vi "AmpScan TestCode2.vi"() -> ()   [LabVIEW 2018]
panel:
  out "Waveform Graph":dbl[](graph)
  in  "MaxAmp":ext
  in  "AuxPulses":ext[](array[numeric])
  in  "Amp":ext[](array[numeric])
  in  "AuxAmp":ext[](array[numeric])
  out "Amp2":ext
  in  "Scan time":ext
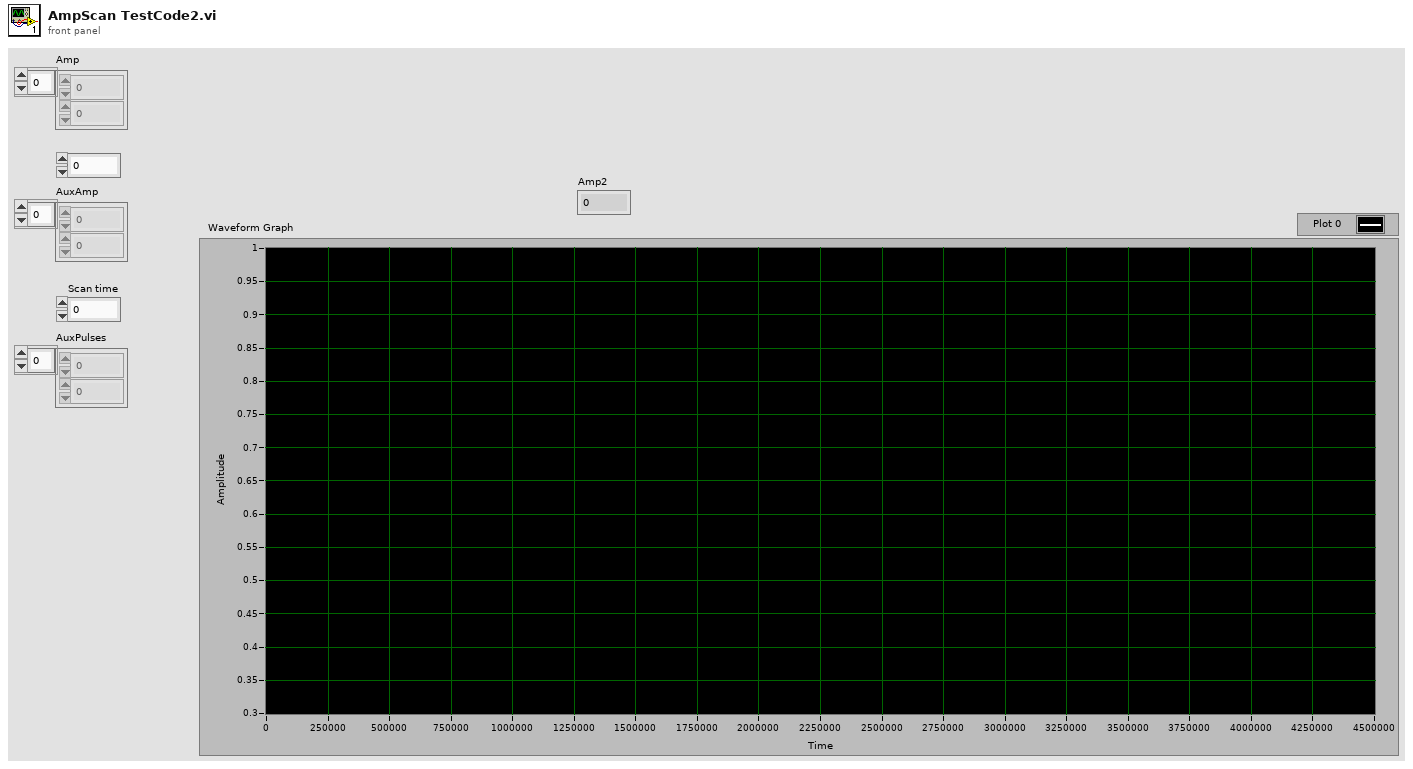
[diagram p1: front panel]
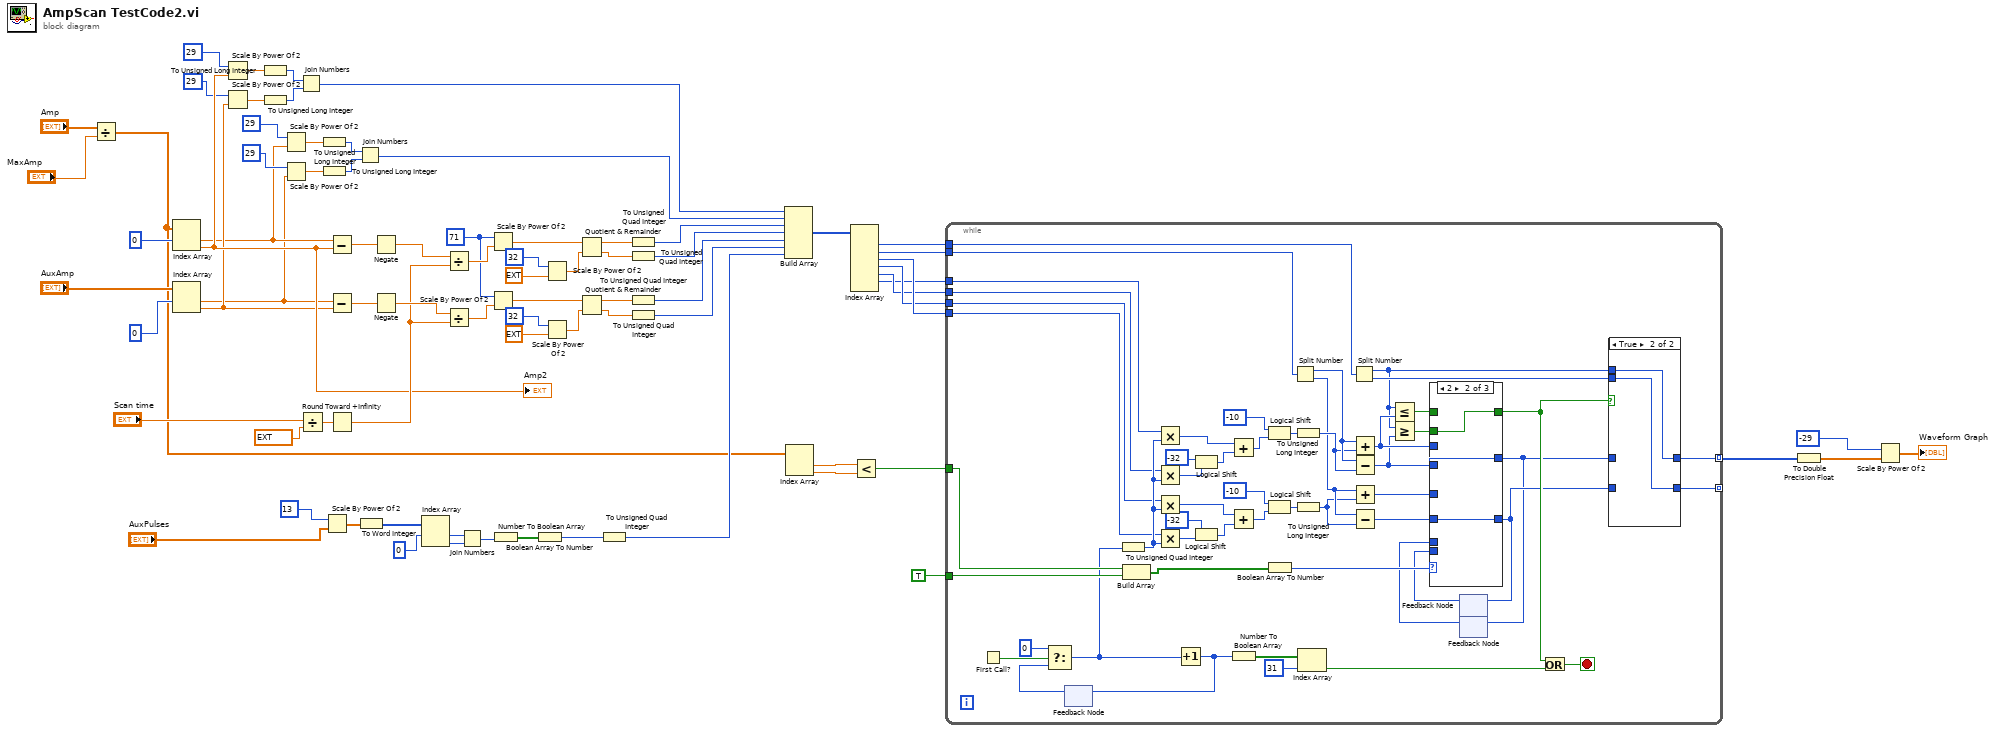
[diagram p0: block diagram]
diagram:
  w65 = i16 71 ("n")
  n1 = Divide(x="Amp", y="MaxAmp") -> (x/y=w7:ext[])
  n2 = Index Array(array=w7, index #1=0 ("index")) -> (element #1=w20:ext, element #2=w33:ext)  [unwired: 1 in]
  "Amp2" <- w33
  n3 = Index Array(array="AuxAmp", index #1=0 ("index")) -> (element #1=w19:ext, element #2=w30:ext)  [unwired: 1 in]
  n4 = Scale By Power Of 2(n=i16 29, x=w33) -> (x*2^n=w61:ext)
  n5 = Scale By Power Of 2(n=i16 29, x=w30) -> (x*2^n=w32:ext)
  n6 = To Unsigned Long Integer(number=w61) -> (unsigned 32bit integer=w29:u32)
  n7 = To Unsigned Long Integer(number=w32) -> (unsigned 32bit integer=w28:u32)
  n8 = Scale By Power Of 2(n=i16 29, x=w20) -> (x*2^n=w22:ext)
  n9 = Scale By Power Of 2(n=i16 29, x=w19) -> (x*2^n=w23:ext)
  n10 = Join Numbers(hi=w29, lo=w28) -> ((hi.lo)=w27:u64)
  n11 = Divide(x="Scan time", y=ext 2.5e-08) -> (x/y=w72:ext)
  n12 = To Unsigned Long Integer(number=w22) -> (unsigned 32bit integer=w25:u32)
  n13 = To Unsigned Long Integer(number=w23) -> (unsigned 32bit integer=w26:u32)
  n14 = Scale By Power Of 2(n=i16 13, x="AuxPulses") -> (x*2^n=w42:ext[])
  n15 = Subtract(x=w20, y=w33) -> (x-y=w77:ext)
  n16 = Subtract(x=w19, y=w30) -> (x-y=w76:ext)
  n17 = Round Toward +Infinity(x=w72) -> (ceil(x): smallest int >= x=w67:ext)
  n18 = Join Numbers(hi=w25, lo=w26) -> ((hi.lo)=w18:u64)
  n19 = To Word Integer(number=w42) -> (16bit integer=w41:i16[])
  n20 = Negate(x=w77) -> (-x=w62:ext)
  n21 = Negate(x=w76) -> (-x=w75:ext)
  n22 = Index Array(array=w41, index #1=0 ("index")) -> (element #1=w39:i16, element #2=w38:i16)  [unwired: 1 in]
  n23 = Divide(x=w62, y=w67) -> (x/y=w66:ext)
  n24 = Divide(x=w75, y=w67) -> (x/y=w64:ext)
  n25 = Join Numbers(hi=w39, lo=w38) -> ((hi.lo)=w37:u32)
  n26 = Scale By Power Of 2(n=w65, x=w66) -> (x*2^n=w57:ext)
  n27 = Scale By Power Of 2(n=w65, x=w64) -> (x*2^n=w53:ext)
  n28 = Number To Boolean Array(number=w37) -> (Boolean array=w36:bool[])
  n29 = Boolean Array To Number(Boolean array=w36) -> (number=w35:u32)
  n30 = Scale By Power Of 2(n=i16 32, x=ext 1.0) -> (x*2^n=w58:ext)
  n31 = Scale By Power Of 2(n=i16 32, x=ext 1.0) -> (x*2^n=w56:ext)
  n32 = Quotient & Remainder(x=w57, y=w58) -> (x-y*floor(x/y)=w52:ext, floor(x/y)=w50:ext)
  n33 = Quotient & Remainder(x=w53, y=w56) -> (x-y*floor(x/y)=w48:ext, floor(x/y)=w46:ext)
  n34 = To Unsigned Quad Integer(1:w35) -> (0:w34:u64)
  n35 = To Unsigned Quad Integer(1:w52) -> (0:w51:u64)
  n36 = To Unsigned Quad Integer(1:w50) -> (0:w49:u64)
  n37 = To Unsigned Quad Integer(1:w48) -> (0:w47:u64)
  n38 = To Unsigned Quad Integer(1:w46) -> (0:w45:u64)
  n39 = Build Array(w27, w18, w51, w49, w47, w45, w34) -> (w17:u64[])
  n40 = Index Array(array=w7) -> (element #1=w9:ext, element #2=w8:ext)  [unwired: 2 in]
  n41 = Index Array(array=w17) -> (element #1=w16:u64, element #2=w15:u64, element #3=w14:u64, element #4=w13:u64, element #5=w12:u64, element #6=w11:u64)  [unwired: 7 in, 1 out]
  n42 = Less?(x=w9, y=w8) -> (x < y?=w6:bool)
  n43 = while {
    tunnel: w16 -> [w91]
    tunnel: w15 -> [w90]
    tunnel: w14 -> [w86]
    tunnel: w13 -> [w87]
    tunnel: w12 -> [w88]
    tunnel: w11 -> [w89]
    tunnel: w6 -> [w93]
    tunnel: TRUE -> [w92]
    tunnel: [w79] -> w2 mode=indexing
    tunnel: [w78] -> _ mode=indexing
    stop <- w123 stop-if-true
    n44 = First Call?() -> (First Call?: T/F=w128:bool)
    n45 = feedback #1() -> (w129:u32)  [unwired: 1 in]
    n46 = Select(t=u32 0 ("index"), s=w128, f=w129) -> (s? t:f=w85:u32)
    n47 = To Unsigned Quad Integer(1:w85) -> (0:w108:u64)
    n48 = Build Array(w93, w92) -> (w103:bool[])
    n49 = Multiply(x=w89, y=w108) -> (x*y=w122:u64)
    n50 = Multiply(x=w88, y=w108) -> (x*y=w120:u64)
    n51 = Multiply(x=w87, y=w108) -> (x*y=w111:u64)
    n52 = Multiply(x=w86, y=w108) -> (x*y=w110:u64)
    n53 = Increment(x=w85) -> (x+1=w127:u32)
    n54 = feedback-in #1(w127) -> ()
    n55 = Logical Shift(y=i16 -32 ("n"), x=w120) -> (x << y=w119:u64)
    n56 = Logical Shift(y=i16 -32 ("n"), x=w110) -> (x << y=w113:u64)
    n57 = Add(x=w122, y=w119) -> (x+y=w117:u64)
    n58 = Add(x=w111, y=w113) -> (x+y=w115:u64)
    n59 = Number To Boolean Array(number=w127) -> (Boolean array=w126:bool[])
    n60 = Logical Shift(y=i16 -10 ("n"), x=w117) -> (x << y=w116:u64)
    n61 = Logical Shift(y=i16 -10 ("n"), x=w115) -> (x << y=w109:u64)
    n62 = Boolean Array To Number(Boolean array=w103) -> (number=w102:u32)
    n63 = Split Number(x=w90) -> (hi(x)=w107:u32, lo(x)=w105:u32)
    n64 = To Unsigned Long Integer(number=w116) -> (unsigned 32bit integer=w106:u32)
    n65 = To Unsigned Long Integer(number=w109) -> (unsigned 32bit integer=w104:u32)
    n66 = Index Array(array=w126, index=31) -> (element=w124:bool)
    n67 = Split Number(x=w91) -> (hi(x)=w80:u32, lo(x)=w81:u32)
    n68 = Add(x=w107, y=w106) -> (x+y=w97:u32)
    n69 = Subtract(x=w107, y=w106) -> (x-y=w96:u32)
    n70 = Add(x=w105, y=w104) -> (x+y=w101:u32)
    n71 = Subtract(x=w105, y=w104) -> (x-y=w100:u32)
    n72 = Less Or Equal?(x=w80, y=w97) -> (x <= y?=w94:bool)
    n73 = Greater Or Equal?(x=w80, y=w96) -> (x >= y?=w95:bool)
    n74 = feedback #2() -> (w99:u32)  [unwired: 1 in]
    n75 = feedback #3() -> (w98:u32)  [unwired: 1 in]
    n76 = case shown="2" w102 {
      tunnel: w97 -> [_ _ w142]
      tunnel: w96 -> [_ w139 _]
      tunnel: w101 -> [_ _ w141]
      tunnel: w100 -> [_ w138 _]
      tunnel: w99 -> [w135 _ _]
      tunnel: [w136 w139 w142] -> w82
      tunnel: [w135 w138 w141] -> w83
      tunnel: w98 -> [w136 _ _]
      tunnel: w95 -> [_ w137 _]
      tunnel: w94 -> [_ _ w140]
      tunnel: [_ w137 w140] -> w84
      frame Default {
      }
      frame 2 {
      }
      frame 3 {
      }
    }
    n77 = feedback-in #2(w83) -> ()
    n78 = feedback-in #3(w82) -> ()
    n79 = Or(x=w84, y=w124) -> (x .or. y?=w123:bool)
    n80 = case shown="True" w84 {
      tunnel: w80 -> [_ w134]
      tunnel: w81 -> [_ w133]
      tunnel: [w132 w134] -> w79
      tunnel: [w131 w133] -> w78
      tunnel: w82 -> [w132 _]
      tunnel: w83 -> [w131 _]
      frame False {
      }
      frame True {
      }
    }
  }
  n81 = To Double Precision Float(number=w2) -> (double precision float=w4:dbl[])
  n82 = Scale By Power Of 2(n=i16 -29, x=w4) -> (x*2^n=→"Waveform Graph":dbl[])
